vi "SpreadsheetRead.vi"() -> ()   [LabVIEW 2015]
uses:
  <vilib>/Utility/file.llb/Read Delimited Spreadsheet (DBL).vi
panel:
  out "XY Graph":cluster{"all rows":dbl[], "all rows":dbl[]}(graph)
  out "Cluster":cluster{"X array":dbl[], "Y Array":dbl[]}
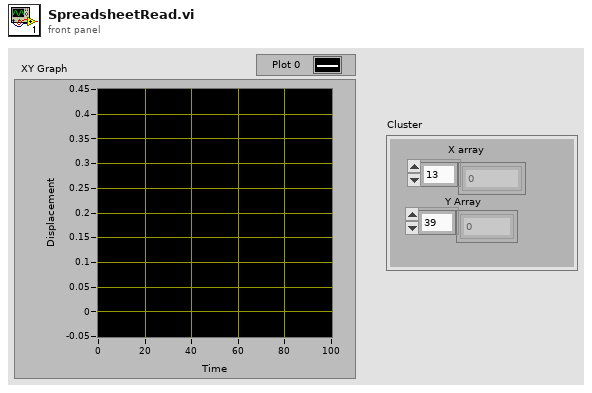
[diagram p1: front panel]
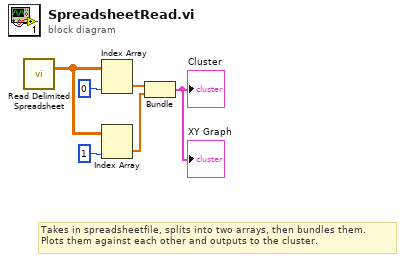
[diagram p0: block diagram]
diagram:
  # "Takes in spreadsheetfile, splits into two arrays, then bundles them.  \nPlots them against each other and outputs to the cluster."
  n1 = call-poly <vilib>:"Read Delimited Spreadsheet.vi"() -> ("all rows"=w5:dbl[][])  [unwired: 10 in, 5 out]
  n2 = Index Array(array=w5, index (col)=0) -> (element=w2:dbl[])  [unwired: 1 in]
  n3 = Index Array(array=w5, index (col)=1) -> (element=w3:dbl[])  [unwired: 1 in]
  n4 = Bundle("all rows"=w2, "all rows"=w3) -> (→"Cluster" →"XY Graph":cluster{"all rows":dbl[], "all rows":dbl[]})  [unwired: 1 in]
